vi "Read Bool1D A.vi"(8 "error in (no error)":errorcluster, 11 "Two Terminal in":refnum<class "AbsFunc_Two Term_Bool_1D.lvclass">) -> (0 "error out":errorcluster, 2 "Abs_Types.lvlib:Boolean.lvclass":refnum<class "Abs_Boolean_1D.lvclass">, 3 "Two Terminal out":refnum<class "AbsFunc_Two Term_Bool_1D.lvclass">)   [LabVIEW 2021, in "AbsFunc_Two Term_Bool_1D.lvclass"]
uses:
  AbsFunc_Two Term_Bool_1D.lvclass
  Abs_Types/Boolean_1D/Abs_Boolean_1D.lvclass
  AbsFunc_Two Term_Bool_1D.lvclass/AbsFunc_Two Term_Bool_1D.ctl
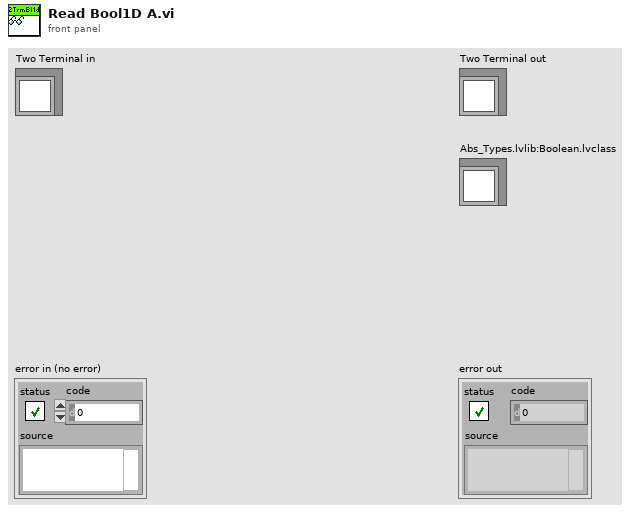
[diagram p1: front panel]
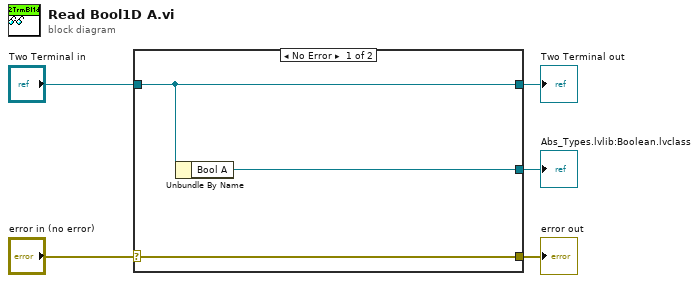
[diagram p0: block diagram]
diagram:
  n1 = case shown="No Error" "error in (no error)" {
    selector: "error in (no error)" -> [w8 w9]
    tunnel: [w8 w9] -> w4
    tunnel: [w7 w10] -> w2
    tunnel: "Two Terminal in" -> [w7 w10]
    tunnel: [w6 _] -> w1
    frame No Error {
      n2 = Unbundle By Name(w7) -> ("Bool A"=w6:refnum<class "Abs_Boolean_1D.lvclass">)
    }
    frame Error {
    }
  }
  "error out" <- w4
  "Two Terminal out" <- w2
  "Abs_Types.lvlib:Boolean.lvclass" <- w1
